vi "Import_Positions.vi"(0 "Boolean":bool) -> ()   [LabVIEW 2013]
panel:
  in  "File Path":path
  out "P10":dbl[](array[numeric])
  out "P9":dbl[](array[numeric])
  out "P8":dbl[](array[numeric])
  out "P6":dbl[](array[numeric])
  out "P5":dbl[](array[numeric])
  out "P4":dbl[](array[numeric])
  out "P7":dbl[](array[numeric])
  out "P3":dbl[](array[numeric])
  out "P2":dbl[](array[numeric])
  out "P1":dbl[](array[numeric])
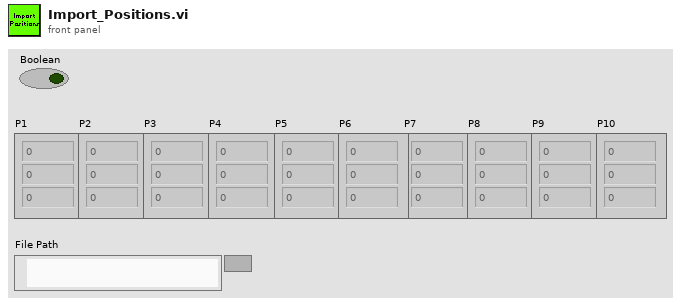
[diagram p1: front panel]
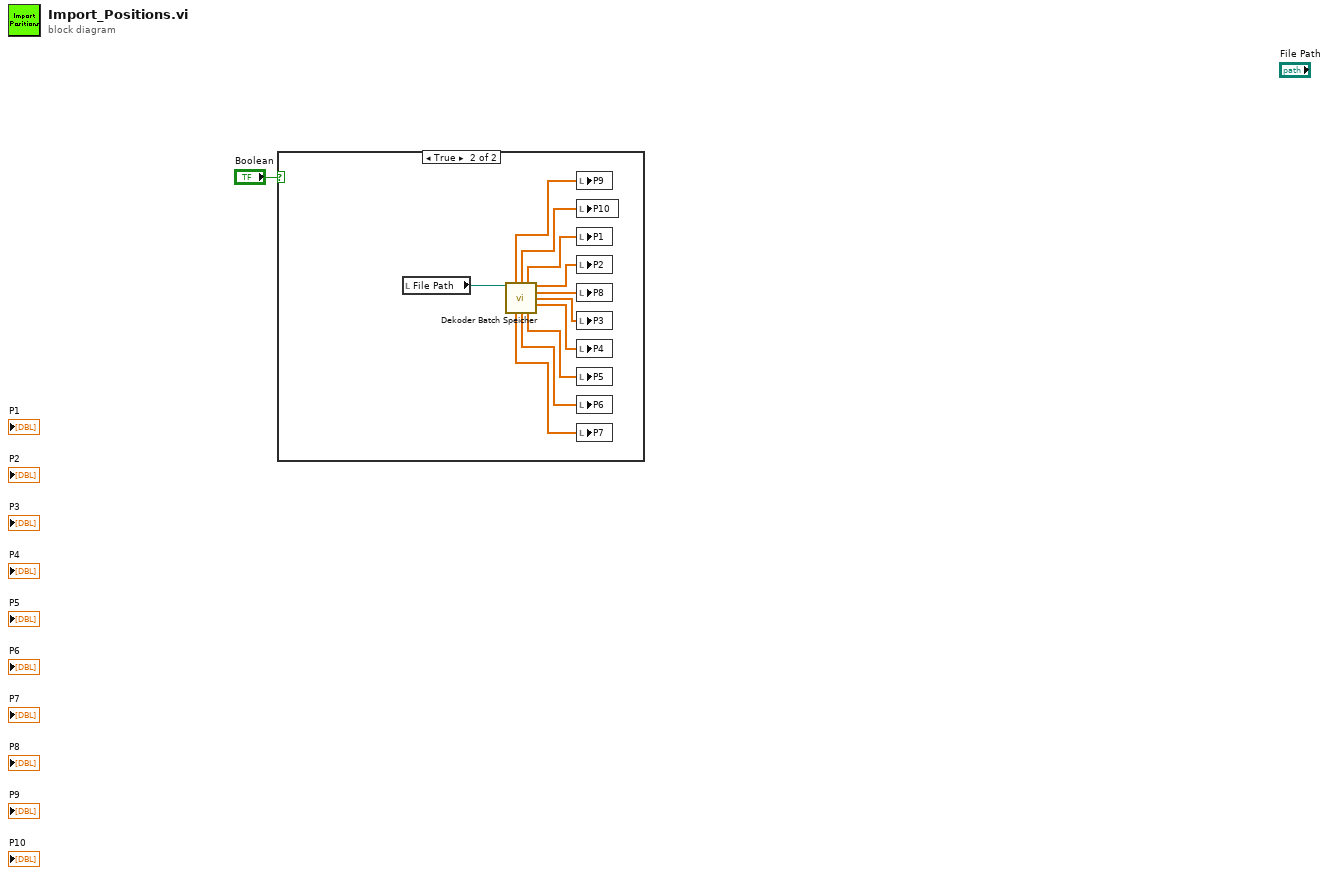
[diagram p0: block diagram]
diagram:
  n1 = case shown="True" "Boolean" {
    frame False {
    }
    frame True {
      n2 = local read "File Path"() -> (w12:path)
      n3 = call "Dekoder Batch Speicher.vi"("Batchfeld Speicher"=w12) -> ("P9"=w2:dbl[], "P10"=w3:dbl[], "P1"=w4:dbl[], "P2"=w5:dbl[], "P8"=w6:dbl[], "P3"=w7:dbl[], "P4"=w8:dbl[], "P7"=w11:dbl[], "P6"=w9:dbl[], "P5"=w10:dbl[])  [unwired: 5 in]
      n4 = local write "P9"(w2) -> ()
      n5 = local write "P10"(w3) -> ()
      n6 = local write "P1"(w4) -> ()
      n7 = local write "P2"(w5) -> ()
      n8 = local write "P8"(w6) -> ()
      n9 = local write "P3"(w7) -> ()
      n10 = local write "P4"(w8) -> ()
      n11 = local write "P5"(w10) -> ()
      n12 = local write "P6"(w9) -> ()
      n13 = local write "P7"(w11) -> ()
    }
  }
